vi "Configure Generator Trigger.vi"(5 "Timeout (1.0)":dbl=1.0 format="%^.3e", 6 "Timeout Enabled (On)":bool=TRUE, 7 "Source (\"Source\")":string="Source", 8 "error in (no error)":errorcluster, 9 "Delay (0.0)":dbl format="%^.3e", 10 "Instance (1)":i32=1, 11 "VISA resource name":refnum<visa-resource-name>) -> (0 "error out":errorcluster, 3 "VISA resource name out":refnum<visa-resource-name>)   [LabVIEW 2020, in "Rohde&Schwarz CMXP GPRF.lvlib"]
doc: "Configures the generator trigger.\n\nAttribute(s):\nRSCMXPGPRF_ATTR_BASEBAND_TRIGGER_SOURCE\nRSCMXPGPRF_ATTR_BASEBAND_TRIGGER_DELAY\nRSCMXPGPRF_ATTR_BASEBAND_TRIGGER_TIMEOUT\nRSCMXPGPRF_ATTR_BASEBAND_TRIGGER_TIMEOUT_ENABLED\n\nRemote-control command(s):\nTRIGger:GPRF:GEN<i>[:ARB]:SOURce\nTRIGger:GPRF:GEN<i>[:ARB]:DELay\nTRIGger:GPRF:GEN<i>:TOUT"
uses:
  <instrlib>/Rohde&Schwarz CMXP GPRF/Rohde&Schwarz CMXP GPRF.lvlib
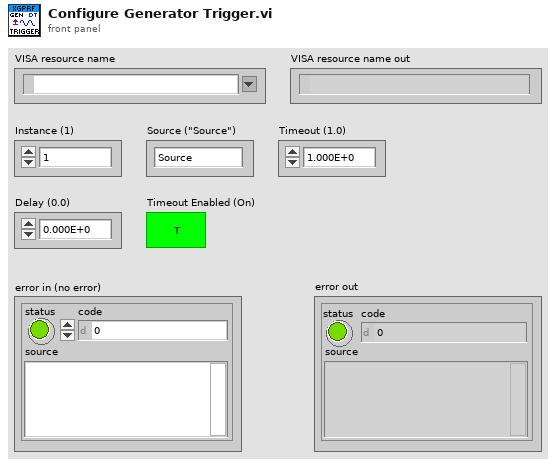
[diagram p1: front panel]
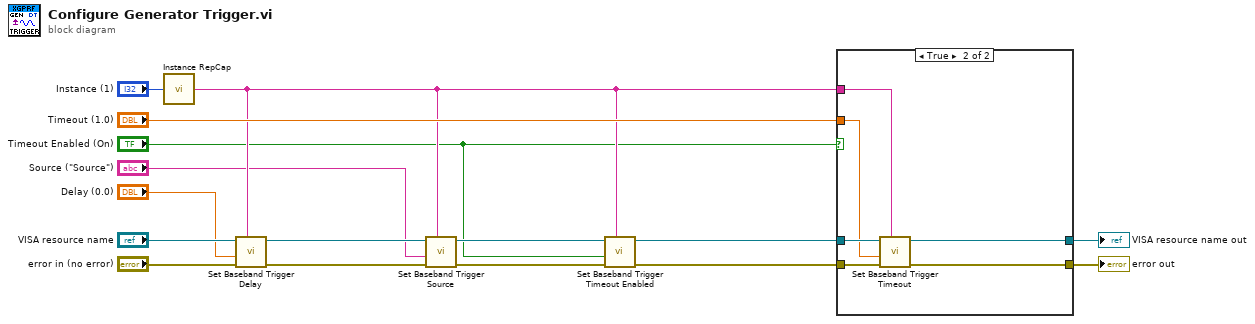
[diagram p0: block diagram]
diagram:
  n1 = call <instrlib>:"Instance RepCap.vi"("Instance in"="Instance (1)") -> ("Instance out"=w5:string)
  n2 = call "Set Baseband Trigger Delay"("Repeated Capabilities"=w5, "error in (no error)"="error in (no error)", "Baseband Trigger Delay (0.0)"="Delay (0.0)", "instrument handle"="VISA resource name") -> ("error out"=w13:errorcluster, "instrument handle out"=w14:refnum<visa-resource-name>)  [unwired: 6 in]
  n3 = call "Set Baseband Trigger Source"("Repeated Capabilities"=w5, "error in (no error)"=w13, "Baseband Trigger Source ()"="Source (\"Source\")", "instrument handle"=w14) -> ("error out"=w11:errorcluster, "instrument handle out"=w12:refnum<visa-resource-name>)  [unwired: 6 in]
  n4 = call "Set Baseband Trigger Timeout Enabled"("Repeated Capabilities"=w5, "error in (no error)"=w11, "Baseband Trigger Timeout Enabled (OFF)"="Timeout Enabled (On)", "instrument handle"=w12) -> ("error out"=w7:errorcluster, "instrument handle out"=w8:refnum<visa-resource-name>)  [unwired: 6 in]
  n5 = case shown="True" "Timeout Enabled (On)" {
    tunnel: [w17 w24] -> w10
    tunnel: [w18 w23] -> w9
    tunnel: w8 -> [w18 w22]
    tunnel: w7 -> [w17 w21]
    tunnel: "Timeout (1.0)" -> [_ w19]
    tunnel: w5 -> [_ w20]
    frame False {
    }
    frame True {
      n6 = call "Set Baseband Trigger Timeout"("Repeated Capabilities"=w20, "error in (no error)"=w21, "Baseband Trigger Timeout (0.0)"=w19, "instrument handle"=w22) -> ("error out"=w24:errorcluster, "instrument handle out"=w23:refnum<visa-resource-name>)  [unwired: 6 in]
    }
  }
  "error out" <- w10
  "VISA resource name out" <- w9
